vi "Alltesta Wait for Idle.vi"(6 "Timeout (s)":dbl=10.0 format="%#_13g", 7 "Poll Command":string="B1?", 8 "error in (no error)":errorcluster, 9 "Lower Bound":i32=-1000000000, 10 "Upper Bound":i32=1000000000, 11 "Serial Port in":refnum<visa-resource-name>="COM3") -> (0 "error out":errorcluster, 3 "Serial Port out":refnum<visa-resource-name>="COM3")   [LabVIEW 2023, in "Alltesta Autosampler.lvlib"]
uses:
  Alltesta Autosampler.lvlib
panel:
  out "Finished?":bool
  out "Status":string
  in  "Poll time (s)":dbl=0.2
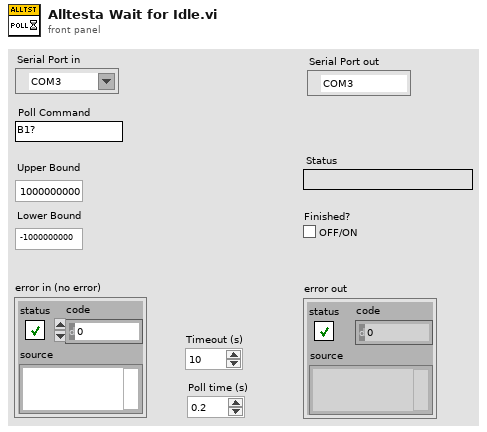
[diagram p1: front panel]
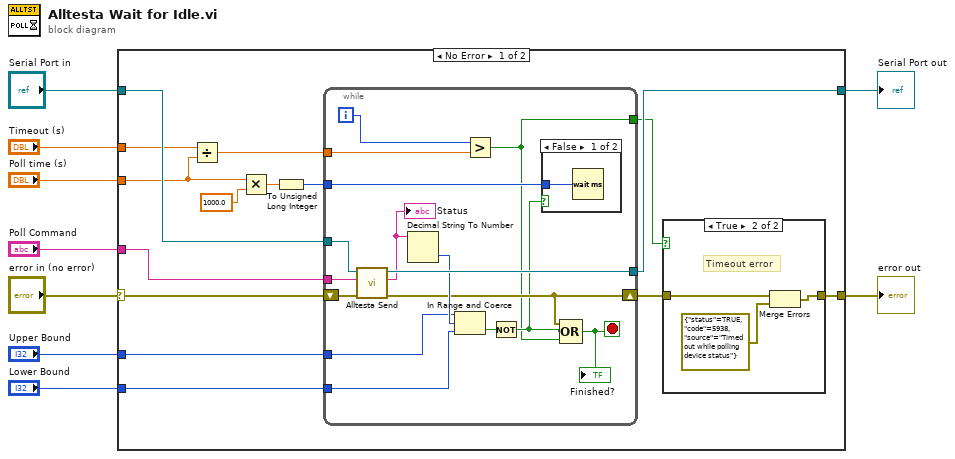
[diagram p0: block diagram]
diagram:
  n1 = case shown="No Error" "error in (no error)" {
    selector: "error in (no error)" -> [w24 w47]
    tunnel: [w12 w47] -> w9
    tunnel: "Serial Port in" -> [w23 w46]
    tunnel: [w17 w46] -> w6
    tunnel: "Timeout (s)" -> [w22 _]
    tunnel: "Poll time (s)" -> [w21 _]
    tunnel: "Poll Command" -> [w16 _]
    tunnel: "Upper Bound" -> [w11 _]
    tunnel: "Lower Bound" -> [w10 _]
    frame No Error {
      n2 = Divide(x=w22, y=w21) -> (x/y=w15:dbl)
      n3 = Multiply(x=w21, y=1000.0) -> (x*y=w19:dbl)
      n4 = To Unsigned Long Integer(number=w19) -> (unsigned 32bit integer=w18:u32)
      n5 = while {
        tunnel: w23 -> [w43]
        tunnel: [w42] -> w17
        shift-right: [w31] -> w13
        shift-left: w24 -> [w44]
        tunnel: w18 -> [w41]
        tunnel: w16 -> [w40]
        tunnel: w11 -> [w37]
        tunnel: w10 -> [w36]
        tunnel: w15 -> [w33]
        tunnel: [w29] -> w14
        i -> [w34]
        stop <- w32 stop-if-true
        n6 = call "Alltesta Send.vi"("error in (no error)"=w44, "Command"=w40, "Serial Port in"=w43) -> ("error out"=w31:errorcluster, "Response"=w39:string, "Serial Port out"=w42:refnum<visa-resource-name>)  [unwired: 6 in]
        "Status" <- w39
        n7 = Decimal String To Number(string=w39) -> (number=w38:i32)  [unwired: 2 in, 1 out]
        n8 = In Range and Coerce(upper limit=w37, x=w38, lower limit=w36) -> (In Range?=w35:bool)  [unwired: 1 out]
        n9 = Greater?(x=w34, y=w33) -> (0:w29:bool)
        n10 = Not(x=w35) -> (.not. x?=w30:bool)
        n11 = case shown="False" w30 {
          tunnel: w41 -> [w45 _]
          frame False {
            n12 = Wait (ms)(milliseconds to wait=w45) -> ()  [unwired: 1 out]
          }
          frame True {
          }
        }
        n13 = Compound Arithmetic op=OR(w31, w30, w29) -> (w32:bool)
        "Finished?" <- w32
      }
      n14 = case shown="True" w14 {
        tunnel: w13 -> [w25 w28]
        tunnel: [w25 w27] -> w12
        frame False {
        }
        frame True {
          # "Timeout error"
          n15 = Merge Errors(w28, errorcluster {"status"=TRUE, "code"=5938, "source"="Timed out while polling device status"} ("error in")) -> (w27:errorcluster)
        }
      }
    }
    frame Error {
    }
  }
  "error out" <- w9
  "Serial Port out" <- w6
